vi "DDC 2945 2955 (Four Channels).vi"(0 "data in":T1[](array[typedef]), 1 "reset":bool, 5 "start trigger":bool, 9 "enable":bool[](array[boolean]), 11 "ddc parameters":T2[](array[typedef]) {"if frequency shift" format="%#.48g"; "frequency shift" format="%#.48g"}) -> (4 "data out":u32[](array[numeric]), 6 "number of overflows":u64[](array[numeric]), 10 "output valid":bool, 14 "dsp reset done":bool)   [LabVIEW 2021]
doc: "Controls whether or not data is written to the DMA FIFO for the acquisition stream. If burst size is 0, this will be a continuous stream, started when the start trigger is asserted. If burst size is greater than zero, acquisition will be in bursts of the designated size, initiated each time the internal state machine is idle and a start trigger is received.\n\nThis VI also keeps track of whether or not an overflow occurred in the acquisition stream and counts the number of overflows that have occurred for debugging information.\n\nThe internal state machine returns the number of samples processed since the most recent acquisition began and the current state machine state."
uses:
  DDC Parameters 2945 2955.ctl
  <instrlib>/_niInstr/DSP/v1/Shared/Public/IQ Impairments.ctl
  <instrlib>/_niInstr/DSP/v1/Shared/Public/IQ Data.ctl
  <instrlib>/_niInstr/DSP/v1/Shared/niInstr DSP v1 Shared.lvlib
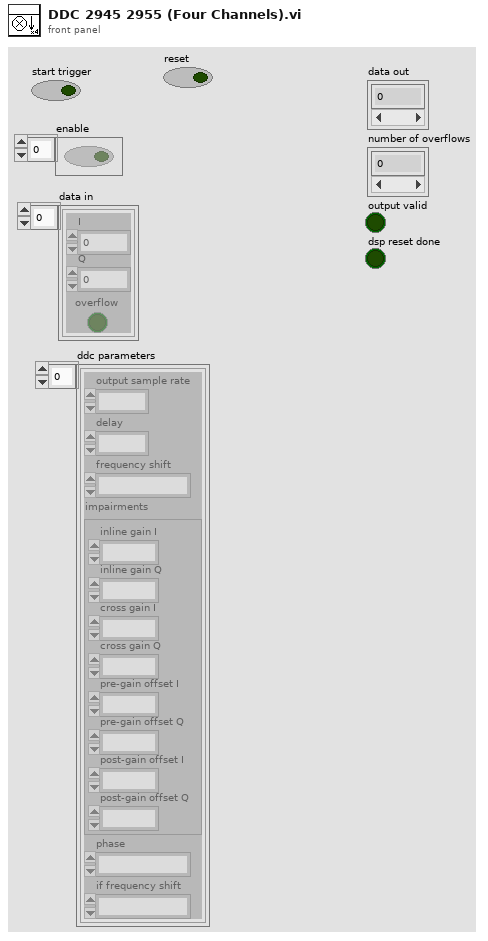
[diagram p1: front panel]
types:
  T1 = typedef "niInstr DSP v1 Shared.lvlib/IQ Data.ctl" = cluster{"I":fxp<+/-,18,1>, "Q":fxp<+/-,18,1>, "overflow":bool}
  T2 = typedef "DDC Parameters 2945 2955.ctl" = cluster{"output sample rate":fxp<+,48,1>, "delay":fxp<+/-,16,0>, "frequency shift":fxp<+/-,48,0>, "impairments":T3, "phase":fxp<+/-,21,0>, "if frequency shift":fxp<+/-,48,0>}
  T3 = typedef "niInstr DSP v1 Shared.lvlib/IQ Impairments.ctl" = cluster{"inline gain I":fxp<+/-,18,1>, "inline gain Q":fxp<+/-,18,1>, "cross gain I":fxp<+/-,18,1>, "cross gain Q":fxp<+/-,18,1>, "pre-gain offset I":fxp<+/-,18,1>, "pre-gain offset Q":fxp<+/-,18,1>, "post-gain offset I":fxp<+/-,18,1>, "post-gain offset Q":fxp<+/-,18,1>}
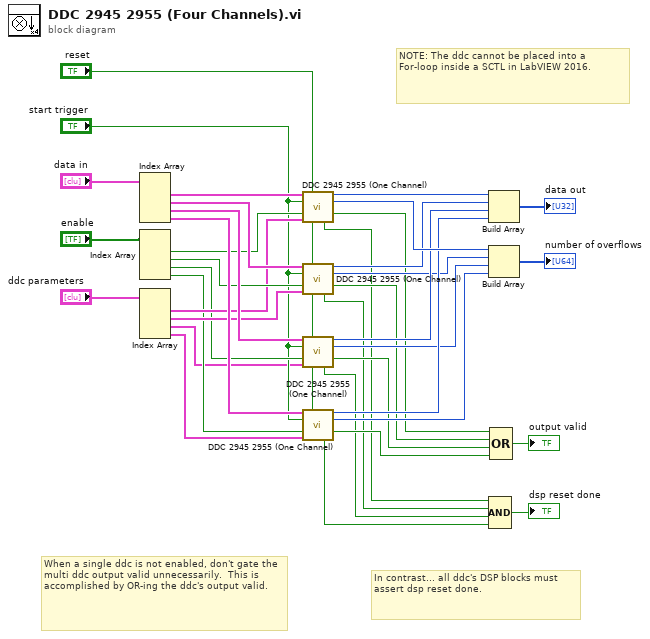
[diagram p0: block diagram]
diagram:
  # "NOTE: The ddc cannot be placed into a For-loop inside a SCTL in LabVIEW 2016."
  # "When a single ddc is not enabled, don't gate the multi ddc output valid unnecessarily.  This is accomplished by OR-ing the ddc's output valid."
  # "In contrast... all ddc's DSP blocks must assert dsp reset done."
  n1 = Index Array(array="data in") -> (element #1=w31:T1, element #2=w28:T1, element #3=w27:T1, element #4=w26:T1)  [unwired: 4 in]
  n2 = Index Array(array="enable") -> (element #1=w25:bool, element #2=w24:bool, element #3=w21:bool, element #4=w20:bool)  [unwired: 4 in]
  n3 = Index Array(array="ddc parameters") -> (element #1=w23:T2, element #2=w22:T2, element #3=w17:T2, element #4=w18:T2)  [unwired: 4 in]
  n4 = call "DDC 2945 2955 (One Channel).vi"("data in"=w31, "reset"="reset", "start trigger"="start trigger", "enable"=w25, "ddc parameters"=w23) -> ("data out"=w30:u32, "number of overflows"=w29:u64, "output valid"=w9:bool, "dsp reset done"=w4:bool)  [unwired: 7 in]
  n5 = call "DDC 2945 2955 (One Channel).vi"("data in"=w28, "reset"="reset", "start trigger"="start trigger", "enable"=w24, "ddc parameters"=w22) -> ("data out"=w15:u32, "number of overflows"=w12:u64, "output valid"=w8:bool, "dsp reset done"=w3:bool)  [unwired: 7 in]
  n6 = call "DDC 2945 2955 (One Channel).vi"("data in"=w27, "reset"="reset", "start trigger"="start trigger", "enable"=w21, "ddc parameters"=w17) -> ("data out"=w14:u32, "number of overflows"=w11:u64, "output valid"=w7:bool, "dsp reset done"=w2:bool)  [unwired: 7 in]
  n7 = call "DDC 2945 2955 (One Channel).vi"("data in"=w26, "reset"="reset", "start trigger"="start trigger", "enable"=w20, "ddc parameters"=w18) -> ("data out"=w13:u32, "number of overflows"=w10:u64, "output valid"=w6:bool, "dsp reset done"=w1:bool)  [unwired: 7 in]
  n8 = Build Array(w30, w15, w14, w13) -> (→"data out":u32[])
  n9 = Build Array(w29, w12, w11, w10) -> (→"number of overflows":u64[])
  n10 = Compound Arithmetic op=AND(w4, w3, w2, w1) -> (→"dsp reset done":bool)
  n11 = Compound Arithmetic op=OR(w9, w8, w7, w6) -> (→"output valid":bool)
